vi "Configure Daughterboard LO Sharing.vi"(0 "niUsrpRio Session in":T2 {"Daughterboard Clock Rate" format="%#.3pHz"; "FPGA Data Clock Rate" format="%#.3pHz"; "Data Clock Rate" format="%#.3pHz"; "Characterization Data"."Frequencies [Hz]" format="%#_6p"; "EEPROM Characterization Header"."Pointer to Device Data Header" format="%x"; "EEPROM Characterization Header"."Checksum" format="%x"; "Device Data Header"."Pointer to Characterization Data" format="%x"; "Device Data Header"."Checksum" format="%x"; "EEPROM Header"."Pointer to User Header" format="%x"; "EEPROM Header"."Pointer to Factory Header" format="%x"; "EEPROM Header"."Product Code" format="%x"; "EEPROM Header"."Checksum" format="%x"}, 1 "scope":string, 11 "error in":errorcluster, 12 "lo config":T1) -> (4 "niUsrpRio Session out":T2 {"Daughterboard Clock Rate" format="%#.3pHz"; "FPGA Data Clock Rate" format="%#.3pHz"; "Data Clock Rate" format="%#.3pHz"; "Characterization Data"."Frequencies [Hz]" format="%#_6p"; "EEPROM Characterization Header"."Pointer to Device Data Header" format="%x"; "EEPROM Characterization Header"."Checksum" format="%x"; "Device Data Header"."Pointer to Characterization Data" format="%x"; "Device Data Header"."Checksum" format="%x"; "EEPROM Header"."Pointer to User Header" format="%x"; "EEPROM Header"."Pointer to Factory Header" format="%x"; "EEPROM Header"."Product Code" format="%x"; "EEPROM Header"."Checksum" format="%x"}, 15 "error out":errorcluster)   [LabVIEW 2020]
uses:
  <instrlib>/niUsrpRio/Config/v1/Host/Public/niUsrpRio Session.ctl
  <instrlib>/_niInstr/Register Bus/v0/Host/Public/Register Bus Session.ctl
  <instrlib>/_niInstr/Register Bus/v0/Host/Private/Session Data.ctl
  <instrlib>/niUsrpRio/Config/v1/Host/Private/DB Queue Reference.ctl
  <instrlib>/niUsrpRio/Config/v1/Host/Private/Daughterboard Data.ctl
  <instrlib>/niUsrpRio/Config/v1/Host/Private/ATR state data.ctl
  <instrlib>/niUsrpRio/Config/v1/Host/Private/Antenna Configuration.ctl
  <instrlib>/niUsrpRio/Config/v1/Host/Private/CPLD Power Mode.ctl
  <instrlib>/niUsrpRio/Config/v1/Host/Public/EEPROM Header.ctl
  <instrlib>/niUsrpRio/Config/v1/Host/Public/EEPROM Device Data Header.ctl
  <instrlib>/niUsrpRio/Config/v1/Host/Public/EEPROM Characterization Header.ctl
  <instrlib>/niUsrpRio/Config/v1/Host/Public/Characterization Data.ctl
  <instrlib>/niUsrpRio/Config/v1/Host/Public/IQ Imbalance.ctl
  <instrlib>/niUsrpRio/Config/v1/Host/Private/LO Source.ctl
  <vilib>/Utility/error.llb/Error Cluster From Error Code.vi
  <vilib>/ErrorRing/Error Ring.xnode
  <instrlib>/niUsrpRio/Config/v1/Host/niUsrpRio Config v1 Host.lvlib
  <instrlib>/_niInstr/Register Bus/v0/Host/niInstr Register Bus v0 Host.lvlib
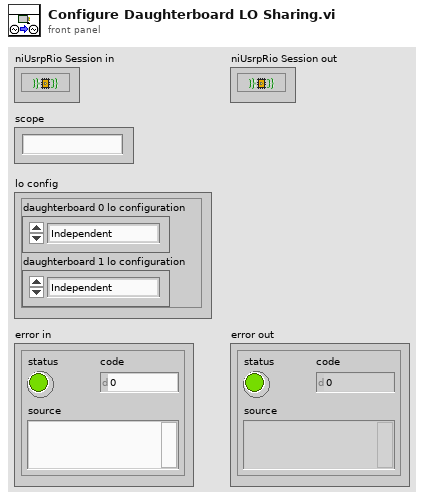
[diagram p1: front panel]
types:
  T1 = cluster{"daughterboard 0 lo configuration":enum16{"Independent", "Import", "Shared and Export", "Reimport", "Shared"}, "daughterboard 1 lo configuration":enum16{"Independent", "Import", "Shared and Export", "Reimport", "Shared"}}
  T2 = typedef "niUsrpRio Config v1 Host.lvlib/niUsrpRio Session.ctl" = cluster{"FPGA Interface":refnum<k20>, "RIO Interface Number":u32, "Data Clock Rate":u32, "FPGA Data Clock Rate":u32, "Global Settings Register Bus":T3, "Radio 0 Settings Register Bus":T3, "Radio 1 Settings Register Bus":T3, "Radio Settings Bus Semaphore":T4, "DB Queues":T5[], "Characterization Data Valid?":bool, "EEPROM Header":T6, "Device Data Header":T7, "EEPROM Characterization Header":T8, "Characterization Data":T9[], "FPGA Current Version":u32, "FPGA Oldest Compatible Version":u32, "Fixed Logic Current Version":u32, "Fixed Logic Oldest Compatible Version":u32, "FPGA Radio Settings Bus Current Version":u32, "FPGA Radio Settings Bus Oldest Compatible Version":u32, "FPGA Board Config Current Version":u32, "FPGA Board Config Oldest Compatible Version":u32, "Daughterboard Clock Rate":u32, "daughterboard configuration session handles":u64[]}
  T3 = typedef "niInstr Register Bus v0 Host.lvlib/Register Bus Session.ctl" = refnum<queue>
  T4 = typedef "Semaphore RefNum" = refnum<k1>
  T5 = typedef "niUsrpRio Config v1 Host.lvlib/DB Queue Reference.ctl" = refnum<queue>
  T6 = typedef "niUsrpRio Config v1 Host.lvlib/EEPROM Header.ctl" = cluster{"Checksum":u32, "Product Code":u16, "Hardware Current Version":u16, "Hardware Oldest Compatible Version":u16, "EEPROM Map Current Version":u16, "EEPROM Map Oldest Compatible Version":u16, "User Password":string, "Pointer to Factory Header":u32, "Pointer to User Header":u32, "Recommended Interval":u16, "Number of Reserved Bytes":i32, "Number of Daughterboards":u8, "Daughterboard IDs":u16[], "Daughterboard Serial Numbers":string[]}
  T7 = typedef "niUsrpRio Config v1 Host.lvlib/EEPROM Device Data Header.ctl" = cluster{"Checksum":u32, "Number of Channels":u8, "Number of Gain Settings":u16[], "Pointer to Characterization Data":u32[], "Number of Reserved Bytes":i32, "Number of Frequencies":u16[]}
  T8 = typedef "niUsrpRio Config v1 Host.lvlib/EEPROM Characterization Header.ctl" = cluster{"Checksum":u32, "Date":timestamp, "Temperature":sgl, "Misc. Info":string, "Pointer to Device Data Header":u32, "Number of Reserved Bytes":i32}
  T9 = typedef "niUsrpRio Config v1 Host.lvlib/Characterization Data.ctl" = cluster{"Gains[dB]":dbl[], "Frequencies [Hz]":dbl[], "IQ Imbalance Table":T10[], "Measured Gains[dB]":dbl[][]}
  T10 = typedef "niUsrpRio Config v1 Host.lvlib/IQ Imbalance.ctl" = cluster{"Gain Imbalance [linear]":dbl, "Phase Imbalance [radians]":dbl, "Offset":cdb}
  T11 = typedef "niUsrpRio Config v1 Host.lvlib/Device Subfunction.ctl" = enum16{"rx", "tx", "all"}
  T12 = typedef "niUsrpRio Config v1 Host.lvlib/DB Types.ctl" = enum16{"sbx", "cbx", "wbx", "unknown", "ubx", "twinrx"}
  T13 = typedef "niUsrpRio Config v1 Host.lvlib/LO Source.ctl" = enum16{"Internal", "Companion", "External", "Reimport"}
  T14 = enum16{"Independent", "Import", "Shared and Export", "Reimport", "Shared"}
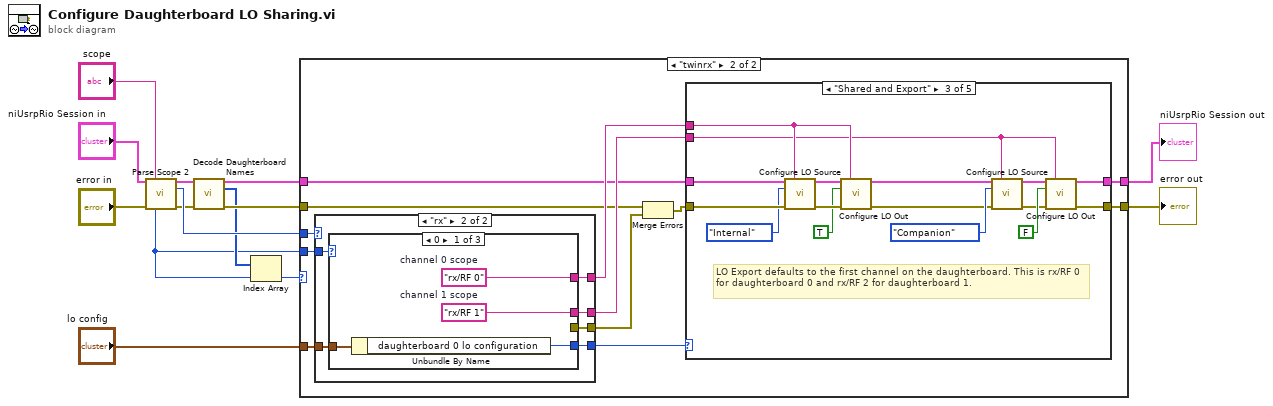
[diagram p0: block diagram]
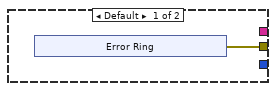
[diagram p3: hidden frame]
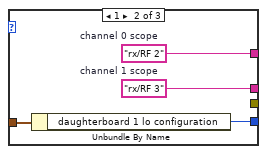
[diagram p4: hidden frame]
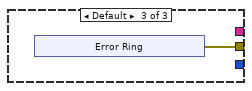
[diagram p5: hidden frame]
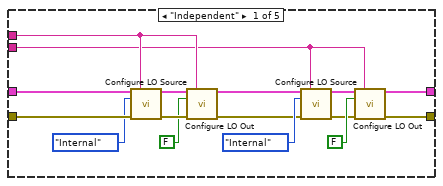
[diagram p6: hidden frame]
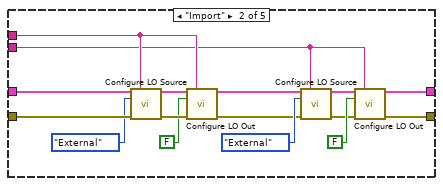
[diagram p7: hidden frame]
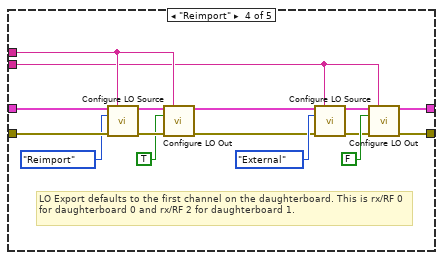
[diagram p8: hidden frame]
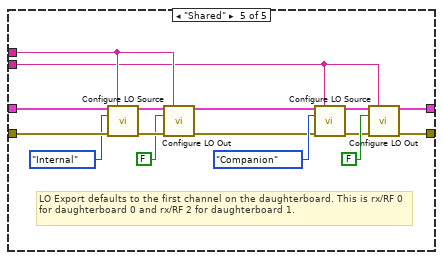
[diagram p9: hidden frame]
diagram:
  n1 = call <instrlib>:"Parse Scope 2.vi"("niUsrpRio Session"="niUsrpRio Session in", "scope"="scope", "error in"="error in") -> ("niUsrpRio Session (out)"=w7:T2, "Device Subfunction"=w8:T11, "daughterboard index"=w2:u32, "error out"=w6:errorcluster)  [unwired: 4 in, 5 out]
  n2 = call <instrlib>:"Decode Daughterboard Names.vi"("niUsrpRio Session"=w7, "error in"=w6) -> ("niUsrpRio Session (out)"=w4:T2, "daughterboard names"=w3:T12[], "error out"=w5:errorcluster)  [unwired: 10 in, 1 out]
  n3 = Index Array(array=w3, index=w2) -> (element=w1:T12)
  n4 = case shown="\"twinrx\"" w1 {
    tunnel: [w15 w23] -> w11
    tunnel: [w16 w22] -> w10
    tunnel: "lo config" -> [_ w21]
    tunnel: w8 -> [_ w20]
    tunnel: w5 -> [w16 w19]
    tunnel: w4 -> [w15 w18]
    tunnel: w2 -> [_ w17]
    frame Default {
    }
    frame "twinrx" {
      n5 = case shown="\"rx\"" w20 {
        tunnel: w17 -> [_ w40]
        tunnel: [_ w39] -> w28
        tunnel: [w29 w38] -> w27
        tunnel: [_ w37] -> w25
        tunnel: [_ w36] -> w24
        tunnel: w21 -> [_ w35]
        frame Default {
          n6 = xnode "Error Ring"() -> ("error out"=w29:errorcluster)
        }
        frame "rx" {
          n7 = case shown="0" w40 {
            tunnel: w35 -> [w44 w48 _]
            tunnel: [w43 w47 _] -> w39
            tunnel: [_ _ w49] -> w38
            tunnel: [w42 w45 _] -> w36
            tunnel: [w41 w46 _] -> w37
            frame 0 {
              w42 = "rx/RF 1"  # channel 1 scope
              w41 = "rx/RF 0"  # channel 0 scope
              n8 = Unbundle By Name(w44) -> ("daughterboard 0 lo configuration"=w43:T14)
            }
            frame 1 {
              w45 = "rx/RF 3"  # channel 1 scope
              w46 = "rx/RF 2"  # channel 0 scope
              n9 = Unbundle By Name(w48) -> ("daughterboard 1 lo configuration"=w47:T14)
            }
            frame Default {
              n10 = xnode "Error Ring"() -> ("error out"=w49:errorcluster)
            }
          }
        }
      }
      n11 = Merge Errors(w19, w27) -> (w26:errorcluster)
      n12 = case shown="\"Shared and Export\"" w28 {
        tunnel: w26 -> [w69 w85 w101 w117 w133]
        tunnel: w18 -> [w70 w86 w102 w118 w134]
        tunnel: w25 -> [w62 w78 w94 w110 w126]
        tunnel: w24 -> [w57 w73 w89 w105 w121]
        tunnel: [w58 w74 w90 w106 w122] -> w23
        tunnel: [w55 w71 w87 w103 w119] -> w22
        frame "Independent" {
          n13 = call <instrlib>:"Configure LO Source.vi"("niUsrpRio Session"=w70, "scope"=w62, "lo source"=LO_Source."Internal", "error in"=w69) -> ("niUsrpRio Session (out)"=w64:T2, "error out"=w68:errorcluster)  [unwired: 10 in]
          n14 = call <instrlib>:"Configure LO Out.vi"("niUsrpRio Session"=w64, "scope"=w62, "enable"=FALSE, "error in"=w68) -> ("niUsrpRio Session (out)"=w63:T2, "error out"=w65:errorcluster)  [unwired: 10 in]
          n15 = call <instrlib>:"Configure LO Source.vi"("niUsrpRio Session"=w63, "scope"=w57, "lo source"=LO_Source."Internal", "error in"=w65) -> ("niUsrpRio Session (out)"=w59:T2, "error out"=w56:errorcluster)  [unwired: 10 in]
          n16 = call <instrlib>:"Configure LO Out.vi"("niUsrpRio Session"=w59, "scope"=w57, "enable"=FALSE, "error in"=w56) -> ("niUsrpRio Session (out)"=w58:T2, "error out"=w55:errorcluster)  [unwired: 10 in]
        }
        frame "Import" {
          n17 = call <instrlib>:"Configure LO Source.vi"("niUsrpRio Session"=w86, "scope"=w78, "lo source"=LO_Source."External", "error in"=w85) -> ("niUsrpRio Session (out)"=w80:T2, "error out"=w84:errorcluster)  [unwired: 10 in]
          n18 = call <instrlib>:"Configure LO Out.vi"("niUsrpRio Session"=w80, "scope"=w78, "enable"=FALSE, "error in"=w84) -> ("niUsrpRio Session (out)"=w79:T2, "error out"=w81:errorcluster)  [unwired: 10 in]
          n19 = call <instrlib>:"Configure LO Source.vi"("niUsrpRio Session"=w79, "scope"=w73, "lo source"=LO_Source."External", "error in"=w81) -> ("niUsrpRio Session (out)"=w75:T2, "error out"=w72:errorcluster)  [unwired: 10 in]
          n20 = call <instrlib>:"Configure LO Out.vi"("niUsrpRio Session"=w75, "scope"=w73, "enable"=FALSE, "error in"=w72) -> ("niUsrpRio Session (out)"=w74:T2, "error out"=w71:errorcluster)  [unwired: 10 in]
        }
        frame "Shared and Export" {
          # "LO Export defaults to the first channel on the daughterboard. This is rx/RF 0 for daughterboard 0 and rx/RF 2 for daughterboard 1."
          n21 = call <instrlib>:"Configure LO Source.vi"("niUsrpRio Session"=w102, "scope"=w94, "lo source"=LO_Source."Internal", "error in"=w101) -> ("niUsrpRio Session (out)"=w96:T2, "error out"=w100:errorcluster)  [unwired: 10 in]
          n22 = call <instrlib>:"Configure LO Out.vi"("niUsrpRio Session"=w96, "scope"=w94, "enable"=TRUE, "error in"=w100) -> ("niUsrpRio Session (out)"=w95:T2, "error out"=w97:errorcluster)  [unwired: 10 in]
          n23 = call <instrlib>:"Configure LO Source.vi"("niUsrpRio Session"=w95, "scope"=w89, "lo source"=LO_Source."Companion", "error in"=w97) -> ("niUsrpRio Session (out)"=w91:T2, "error out"=w88:errorcluster)  [unwired: 10 in]
          n24 = call <instrlib>:"Configure LO Out.vi"("niUsrpRio Session"=w91, "scope"=w89, "enable"=FALSE, "error in"=w88) -> ("niUsrpRio Session (out)"=w90:T2, "error out"=w87:errorcluster)  [unwired: 10 in]
        }
        frame "Reimport" {
          # "LO Export defaults to the first channel on the daughterboard. This is rx/RF 0 for daughterboard 0 and rx/RF 2 for daughterboard 1."
          n25 = call <instrlib>:"Configure LO Source.vi"("niUsrpRio Session"=w118, "scope"=w110, "lo source"=LO_Source."Reimport", "error in"=w117) -> ("niUsrpRio Session (out)"=w112:T2, "error out"=w116:errorcluster)  [unwired: 10 in]
          n26 = call <instrlib>:"Configure LO Out.vi"("niUsrpRio Session"=w112, "scope"=w110, "enable"=TRUE, "error in"=w116) -> ("niUsrpRio Session (out)"=w111:T2, "error out"=w113:errorcluster)  [unwired: 10 in]
          n27 = call <instrlib>:"Configure LO Source.vi"("niUsrpRio Session"=w111, "scope"=w105, "lo source"=LO_Source."External", "error in"=w113) -> ("niUsrpRio Session (out)"=w107:T2, "error out"=w104:errorcluster)  [unwired: 10 in]
          n28 = call <instrlib>:"Configure LO Out.vi"("niUsrpRio Session"=w107, "scope"=w105, "enable"=FALSE, "error in"=w104) -> ("niUsrpRio Session (out)"=w106:T2, "error out"=w103:errorcluster)  [unwired: 10 in]
        }
        frame "Shared" {
          # "LO Export defaults to the first channel on the daughterboard. This is rx/RF 0 for daughterboard 0 and rx/RF 2 for daughterboard 1."
          n29 = call <instrlib>:"Configure LO Source.vi"("niUsrpRio Session"=w134, "scope"=w126, "lo source"=LO_Source."Internal", "error in"=w133) -> ("niUsrpRio Session (out)"=w128:T2, "error out"=w132:errorcluster)  [unwired: 10 in]
          n30 = call <instrlib>:"Configure LO Out.vi"("niUsrpRio Session"=w128, "scope"=w126, "enable"=FALSE, "error in"=w132) -> ("niUsrpRio Session (out)"=w127:T2, "error out"=w129:errorcluster)  [unwired: 10 in]
          n31 = call <instrlib>:"Configure LO Source.vi"("niUsrpRio Session"=w127, "scope"=w121, "lo source"=LO_Source."Companion", "error in"=w129) -> ("niUsrpRio Session (out)"=w123:T2, "error out"=w120:errorcluster)  [unwired: 10 in]
          n32 = call <instrlib>:"Configure LO Out.vi"("niUsrpRio Session"=w123, "scope"=w121, "enable"=FALSE, "error in"=w120) -> ("niUsrpRio Session (out)"=w122:T2, "error out"=w119:errorcluster)  [unwired: 10 in]
        }
      }
    }
  }
  "niUsrpRio Session out" <- w11
  "error out" <- w10
